vi "Parse JSON String.vi"   [LabVIEW 2015, in "JSON.lvlib"]
uses:
  JSON.lvlib
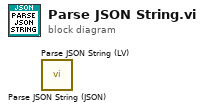
[diagram p0: block diagram]
diagram:
  n1 = call "Parse JSON String (JSON).vi"() -> ()  [unwired: 10 in, 2 out]
  n2 = call "Parse JSON String (LV).vi"() -> ()  [unwired: 10 in, 2 out]
